vi "Loop filter.vi"(7 "e":dbl) -> (6 "a":dbl, 10 "b":dbl)   [LabVIEW 2017]
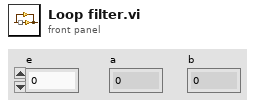
[diagram p1: front panel]
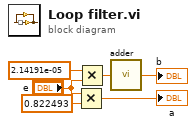
[diagram p0: block diagram]
diagram:
  n1 = Multiply(x="e", y=0.822493) -> (x*y=→"a":dbl)
  n2 = Multiply(x=2.14191e-05, y="e") -> (x*y=w5:dbl)
  n3 = call "adder.vi"("x"=w5) -> ("sum"=→"b":dbl)  [unwired: 14 in]
